vi "RS232 open port.vi"(4 "error in (no error)":errorcluster, 7 "VISA resource name":refnum<visa-resource-name>) -> (0 "error out":errorcluster, 3 "dup VISA resource name":refnum<visa-resource-name>)   [LabVIEW 2016]
uses:
  <vilib>/Instr/_visa.llb/Select Event Type.ctl
  <vilib>/Instr/_visa.llb/VISA Configure Serial Port (Instr).vi
panel:
  in  "baud rate (115200)":u32=115200
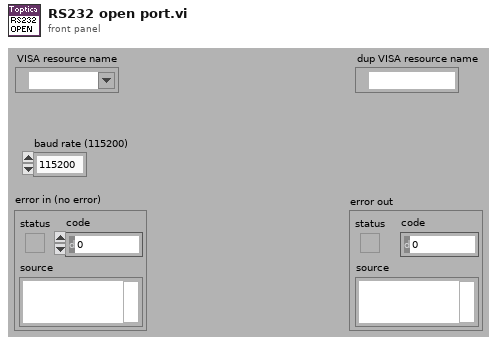
[diagram p1: front panel]
types:
  T1 = typedef "Select Event Type.ctl" = u32
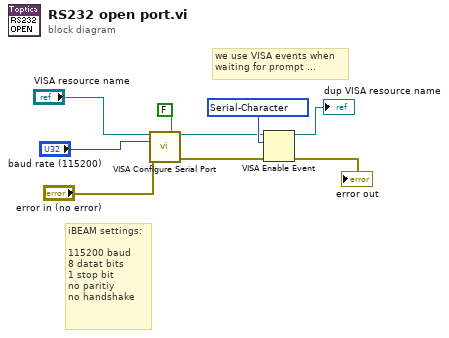
[diagram p0: block diagram]
diagram:
  w8 = T1 1073684533 items=["ServiceRequest"=1073684491, "Trigger"=3221168138, "Clear"=1073684493, "VXI-Signal"=1073684512, "VXI/VME-Interrupt"=3221168161, "VXI/VME-Sysfail"=1073684509, "VXI/VME-Sysreset"=1073684510, "GPIB-CIC"=1073684498, "GPIB-Talk"=1073684499, "GPIB-Listen"=1073684500, "PXI-Interrupt"=1073684514, "Serial-Break"=1073684515, "Serial-TermChar"=1073684516, "Serial-CTS"=1073684521, "Serial-DSR"=1073684522, "Serial-DCD"=1073684524, "Serial-RI"=1073684526, "Serial-Character"=1073684533, "USB-Interrupt"=1073684535, "AllEnabled"=1073709055] ("Event Type")
  # "we use VISA events when\nwaiting for prompt ..."
  # "iBEAM settings:\n\n115200 baud\n8 datat bits\n1 stop bit\nno paritiy\nno handshake"
  n1 = call-poly "VISA Configure Serial Port"("VISA resource name"="VISA resource name", "Enable Termination\nChar (T)"=FALSE ("Enable Termination\nChar (T)"), "baud rate (9600)"="baud rate (115200)", "error in (no error)"="error in (no error)") -> ("VISA resource name out"=w7:refnum<visa-resource-name>, "error out"=w6:errorcluster)  [unwired: 10 in]
  n2 = VISA Enable Event(8:w6, 10:w8, 11:w7) -> (0:→"error out":errorcluster, 3:→"dup VISA resource name":refnum<visa-resource-name>)  [unwired: 1 in]
